vi "GetSpriteActive.vi"(8 "error in (no error)":errorcluster, 10 "Index":i16, 11 "Game in":refnum<class "Game.lvclass">) -> (0 "error out":errorcluster, 2 "Active?":bool, 3 "Game out":refnum<class "Game.lvclass">)   [LabVIEW 2019, in "RT_Game.lvlib" / "Game.lvclass"]
uses:
  Game.lvclass
  Game.lvclass/Game.ctl
  GameObject/GameObject.lvclass/GameObject.ctl
  GameObject/Read IsActive.vi
  RT_Sprite/RT_Sprite.lvclass
  C:/Users/FreshBob/Dropbox/VIs/myRIO_GameConsole/RT/RT_Game/GameObject/GameObject.lvclass
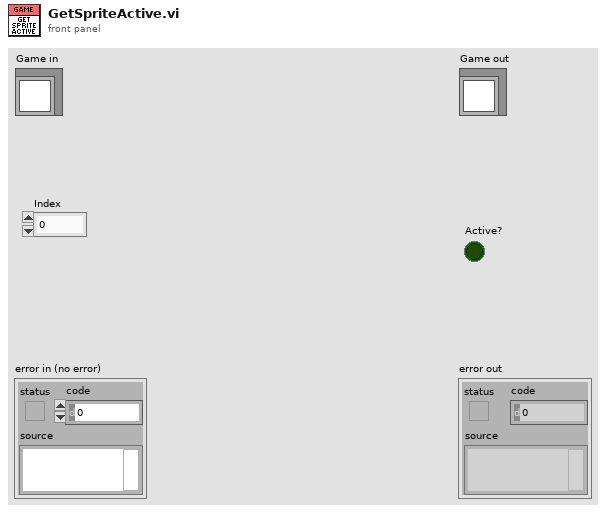
[diagram p1: front panel]
types:
  T1 = typedef "RT_Game.lvlib/Game.lvclass/SpritesCluster.ctl" = cluster{"Sprite1":refnum<class "RT_Sprite.lvclass">, "Sprite2":refnum<class "RT_Sprite.lvclass">, "Sprite3":refnum<class "RT_Sprite.lvclass">}
  T2 = cluster{"Sprites[0]":refnum<class "RT_Sprite.lvclass">, "Sprites[1]":refnum<class "RT_Sprite.lvclass">, "Sprites[2]":refnum<class "RT_Sprite.lvclass">}
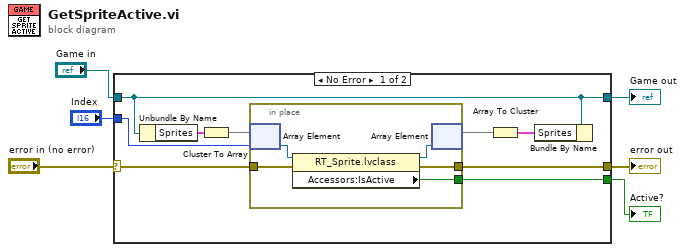
[diagram p0: block diagram]
diagram:
  n1 = case shown="No Error" "error in (no error)" {
    selector: "error in (no error)" -> [w11 w22]
    tunnel: [w10 w22] -> w5
    tunnel: [w13 w21] -> w3
    tunnel: "Game in" -> [w13 w21]
    tunnel: "Index" -> [w12 _]
    tunnel: [w9 _] -> w1
    frame No Error {
      n2 = Unbundle By Name(w13) -> ("Sprites"=w14:T1)
      n3 = Cluster To Array(cluster=w14) -> (array=w8:refnum<class "RT_Sprite.lvclass">[])
      n4 = in-place {
        in-place-border: [w19] -> w10
        in-place-border: w11 -> [w20]
        in-place-border: [w16] -> w9
        n5 = in-place-array #1(w8, w12) -> (w18:refnum<class "RT_Sprite.lvclass">)
        n6 = property class="RT_Sprite.lvclass"(reference=w18, error in=w20) -> (reference out=w17:refnum<class "RT_Sprite.lvclass">, error out=w19:errorcluster, "Accessors:IsActive"=w16:bool)
        n7 = in-place-array #1(w17) -> (w15:refnum<class "RT_Sprite.lvclass">[])  [unwired: 1 out]
      }
      n8 = Array To Cluster(array=w15) -> (cluster=w7:T2)
      n9 = Bundle By Name(cluster=w13, "Sprites"=w7) -> ()  [unwired: 1 out]
    }
    frame Error {
    }
  }
  "error out" <- w5
  "Game out" <- w3
  "Active?" <- w1
